vi "Calculator-V1.1.vi"() -> ()   [LabVIEW 2014]
panel:
  in  "Operator":i32
  out "Result":cluster{dbl}
  in  "y":dbl
  in  "x":dbl
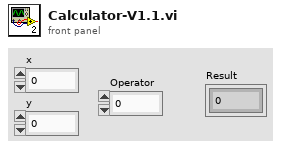
[diagram p1: front panel]
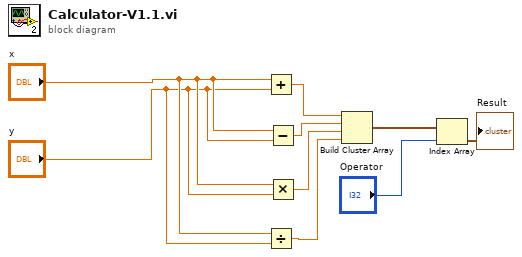
[diagram p0: block diagram]
diagram:
  n1 = Add(x="x", y="y") -> (x+y=w7:dbl)
  n2 = Divide(x="x", y="y") -> (x/y=w4:dbl)
  n3 = Subtract(x="x", y="y") -> (x-y=w6:dbl)
  n4 = Multiply(x="x", y="y") -> (x*y=w5:dbl)
  n5 = Build Cluster Array(w7, w6, w5, w4) -> (w3:cluster{dbl}[])
  n6 = Index Array(array=w3, index="Operator") -> (element=→"Result":cluster{dbl})
